vi "class_data.vi"() -> ()   [LabVIEW 2010, in "GenericImagingMode.lvclass"]
uses:
  GenericImagingMode.lvclass
panel:
  in  "latest instance":refnum<class "GenericImagingMode.lvclass">
  in  "locked by":string
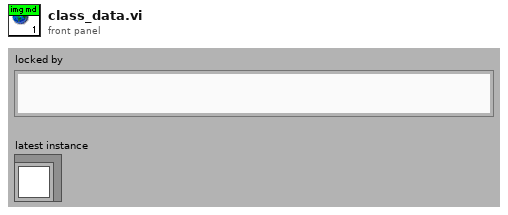
[diagram p1: front panel]
diagram:
